vi "YOLOv8_Pose_OpenVINO.vi"() -> ()   [LabVIEW 2018]
doc: "YOLOv8_Pose_OpenVINO: This example is an example of object detection and pose estimation for the YOLOv8 algorithm. This example calls the models of the object detector and pose estimator, which can simultaneously achieve object detection and human pose estimation. This example combines the target detection performance and pose estimation techniques of the YOLO series, enabling fast and accurate detection of objects and estimation of human pose in images or videos."
uses:
  vi.lib/VIRobotics/ModelZoo/Object_Detection/yolov8_pose_openvino/InitialModel_yolov8_pose_OpenVINO.vi
  vi.lib/VIRobotics/opencv_yiku/Cap/Cap.lvclass
  vi.lib/VIRobotics/ModelZoo/Object_Detection/yolov8_pose_openvino/yolov8_pose_openvino.lvclass
  vi.lib/VIRobotics/opencv_yiku/Mat/Mat_8U/Mat_8U.lvclass
panel:
  in  "device_name":string(combo)="CPU"
  out "每帧耗时(s)":dbl
  in  "class_names_path":path=path "C:/ProgramData/VIRobotics/ModelZoo/Object_Detection/coco.names"
  in  "model_path":path=path "C:/ProgramData/VIRobotics/ModelZoo/Object_Detection/yolov8_pose/onnx_model/yolov8n-pose.onnx"
  in  "stop":bool
  out "picture":picture
  # "Overview: Demonstrates how to use OpenVINO to load the the ONNX model of yolov8-pose for real-time pose detection .\nRequirements: Windows.\nMake sure your computer has a camera。\nInstructions: \n1.Select the device_name to use.（If your computer has Intel GPU, you can select GPU in the \"type\" control before running the VI to achieve faster inference).\n2.Specify the model_file and class_names_file.\n3.Run the VI."
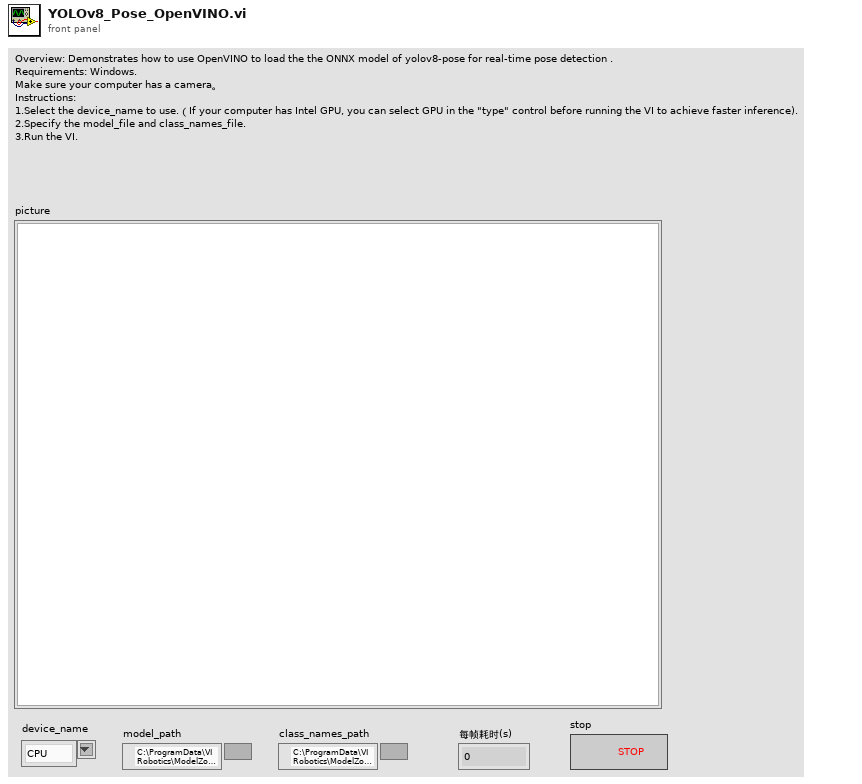
[diagram p1: front panel]
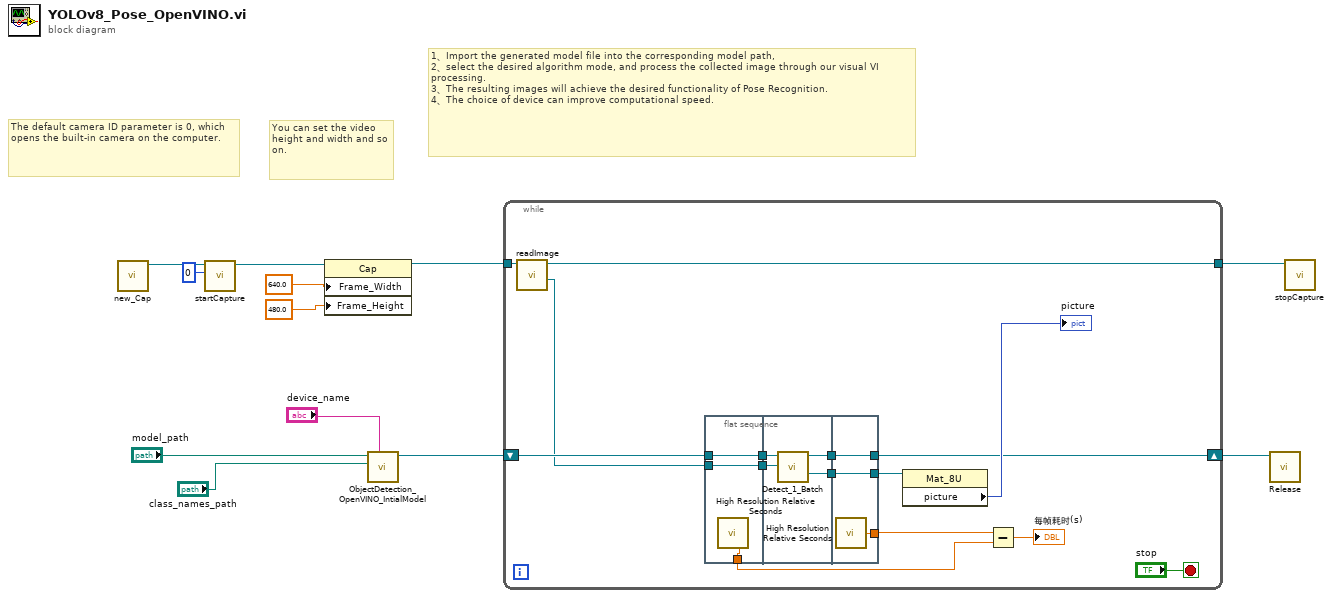
[diagram p0: block diagram]
diagram:
  # "1、Import the generated model file into the corresponding model path, \n2、select the desired algorithm mode, and process the collected image through our visual VI processing. \n3、The resulting images will achieve the desired functionality of Pose Recognition. \n4、The choice of device can improve computational speed."
  # "You can set the video height and width and so on."
  # "The default camera ID parameter is 0, which opens the built-in camera on the computer."
  n1 = call "new_Cap.vi"() -> ("Cap out"=w7:refnum<class "Cap.lvclass">)  [unwired: 10 in, 1 out]
  n2 = call "startCapture.vi"("cameraID"=0, "Cap in"=w7) -> ("Cap out"=w4:refnum<class "Cap.lvclass">)  [unwired: 8 in, 1 out]
  n3 = property class="Cap"(reference=w4, "Frame_Width"=640.0, "Frame_Height"=480.0) -> (reference out=w2:refnum<class "Cap.lvclass">)  [unwired: 1 in, 1 out]
  n4 = call-poly "ObjectDetection_OpenVINO_IntialModel.vi"("device_name"="device_name", "class_names_path"="class_names_path", "path"="model_path") -> ("yolov8_pose_OV out"=w10:refnum<class "yolov8_pose_openvino.lvclass">)  [unwired: 7 in, 1 out]
  n5 = while {
    tunnel: w2 -> [w26]
    shift-right: [w22] -> w11
    shift-left: w10 -> [w27]
    tunnel: [w21] -> w12
    stop <- "stop" stop-if-true
    n6 = call "readImage.vi"("Cap in"=w26) -> ("Mat out"=w14:refnum<class "Mat_8U.lvclass">, "Cap out"=w21:refnum<class "Cap.lvclass">)  [unwired: 8 in, 1 out]
    n7 = flat-sequence {
      tunnel: w27 -> [w30]
      tunnel: [w30] -> w20
      tunnel: [w29] -> w16
      tunnel: w14 -> [w28]
      tunnel: [w28] -> w13
      tunnel: w20 -> [w34]
      tunnel: [w33] -> w19
      tunnel: [w32] -> w18
      tunnel: w13 -> [w31]
      tunnel: [w36] -> w22
      tunnel: [w37] -> w25
      tunnel: w19 -> [w37]
      tunnel: w18 -> [w36]
      tunnel: [w35] -> w17
      frame #0 {
        n8 = call <vilib>:"High Resolution Relative Seconds.vi"() -> ("relative seconds"=w29:dbl)
      }
      frame #1 {
        n9 = call-dynamic "Detect_1_Batch.vi"("image"=w31, "yolov8_pose_openvino in"=w34) -> ("img out"=w33:refnum<class "Mat_8U.lvclass">, "yolov8_pose_openvino out"=w32:refnum<class "yolov8_pose_openvino.lvclass">)  [unwired: 6 in, 2 out]
      }
      frame #2 {
        n10 = call <vilib>:"High Resolution Relative Seconds.vi"() -> ("relative seconds"=w35:dbl)
      }
    }
    n11 = property class="Mat_8U"(reference=w25) -> ("picture"=→"picture":picture)  [unwired: 1 in, 2 out]
    n12 = Subtract(x=w17, y=w16) -> (x-y=→"每帧耗时(s)":dbl)
  }
  n13 = call-dynamic "Release.vi"("yolov8_pose_openvino in"=w11) -> ()  [unwired: 9 in, 2 out]
  n14 = call "stopCapture.vi"("Cap in"=w12) -> ()  [unwired: 10 in, 1 out]
